vi "Destroy.vi"(8 "error in (no error)":errorcluster, 11 "CallHandler in":refnum<class "PyObject.lvclass">) -> (0 "error out":errorcluster, 3 "CallHandler out":refnum<class "PyObject.lvclass">)   [LabVIEW 2013, in "JKI_Python_Bridge_for_LV.lvlib" / "PyObject.lvclass"]
uses:
  PyObject.lvclass
  PyObject.lvclass/PyObject.ctl
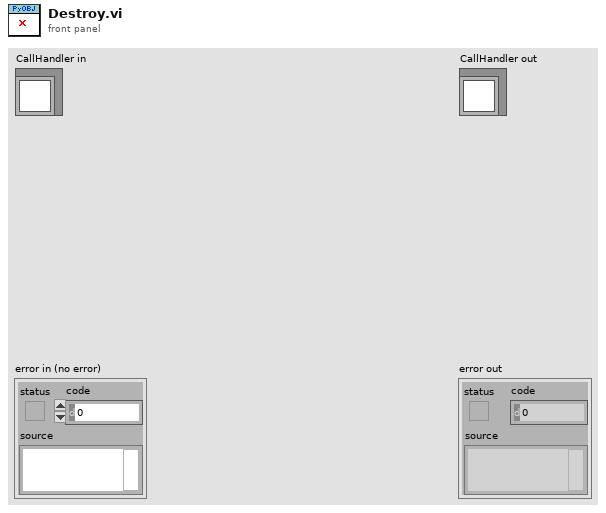
[diagram p1: front panel]
types:
  T1 = typedef "JKI_Python_Bridge_for_LV.lvlib/Server.lvclass/Python Method Call - Event Registration.ctl" = refnum<event-registration>
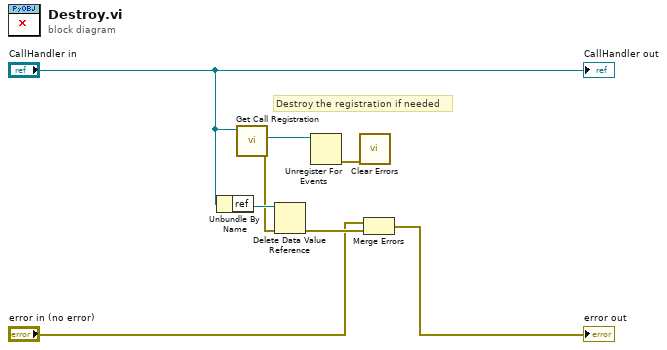
[diagram p0: block diagram]
diagram:
  # "Destroy the registration if needed"
  n1 = Unbundle By Name("CallHandler in") -> ("ref"=w8:refnum<data-value>)
  n2 = call "Get Call Registration.vi"("Node in"="CallHandler in") -> ("error out"=w3:errorcluster, "Call Registration"=w2:T1)  [unwired: 8 in, 1 out]
  n3 = Delete Data Value Reference(data value reference=w8, error in=w3) -> (error out=w7:errorcluster)  [unwired: 1 out]
  n4 = Unregister For Events(event registration refnum=w2) -> (error out=w1:errorcluster)  [unwired: 1 in]
  n5 = call <vilib>:"Clear Errors.vi"("error in (no error)"=w1) -> ()  [unwired: 6 in, 1 out]
  n6 = Merge Errors("error in (no error)", w7) -> (→"error out":errorcluster)
  "CallHandler out" <- "CallHandler in"
